vi "test_Set and Get 9475.vi"(8 "error in (no error)":errorcluster, 11 "TestCase in":refnum<class "Scan Engine Scripting API Custom Device Unit Tests.lvclass">) -> (0 "error out":errorcluster, 3 "TestCase out":refnum<class "Scan Engine Scripting API Custom Device Unit Tests.lvclass">)   [LabVIEW 2020, in "Scan Engine Scripting API Custom Device Unit Tests.lvclass"]
uses:
  Scan Engine Scripting API Custom Device Unit Tests.lvclass
  Scan Engine Scripting API Custom Device Unit Tests.lvclass/Scan Engine Scripting API Custom Device Unit Tests.ctl
  5525f2fe-c77f-4c69-8da2-db807206c7d6.vi
  Shared/Utility/Set Error.vi
  <vilib>/Utility/error.llb/Clear Errors.vi
  Scripting/Utility/Convert Slot Configuration to 9212.vi
  Scripting/Utility/Convert Slot Configuration to 9213.vi
  Scripting/Modules/NI 9475/NI 9475.lvclass
  C:/Users/nitest/Desktop/Git 2020/niveristand-scan-engine-ethercat-custom-device/Custom Device Source/Scripting/Modules/Module/Module.lvclass
  Includes/Modules.lvlibp/SD Module/SD Module.lvclass
  C:/Users/nitest/Desktop/Git 2020/niveristand-scan-engine-ethercat-custom-device/Includes/Modules.lvlibp/RSI Module/RSI Module.lvclass
  Scripting/Modules/NI 9212/NI 9212.lvclass
  Scripting/Modules/NI 9213/NI 9213.lvclass
  Scripting/Modules/NI 9224/NI 9224.lvclass
  Scripting/Modules/NI 9228/NI 9228.lvclass
  Includes/Modules.lvlibp/RSI Module/Read Module Page Property.vi
  Includes/Modules.lvlibp/RSI Module/Read Model.vi
  Scripting/Utility/Convert Module Model to Module Class.vi
  Includes/Modules.lvlibp/SD Module/Read DIO mode.vi
  Includes/Modules.lvlibp/RSI Module/Read Channels.vi
  Scripting/Utility/Convert to DI Module.vi
  Scripting/Utility/Convert to DO Module.vi
  Scripting/Utility/Convert to CI PWM Module.vi
  Scripting/Utility/Convert to CDO Module.vi
  Scripting/Utility/Convert to PWM Module.vi
  Shared/Globals/Error Strings.vi
  Scripting/Utility/Get Channel Names and Default Values for Slot.vi
  Scripting/Modules/NI 9212/Create NI 9212.vi
  Scripting/Modules/NI 9213/Create NI 9213.vi
  Scripting/Utility/Convert to AI Module.vi
  Scripting/Utility/Convert to AI Vrms Module.vi
  Scripting/Utility/Convert to AI Arms Module.vi
  Scripting/Utility/Convert to DIO Module.vi
  Scripting/Modules/Module/Module.lvclass
  Includes/Modules.lvlibp/9212/9212.lvclass
  Includes/Modules.lvlibp/9213/9213.lvclass
  Includes/Modules.lvlibp/9224/9224.lvclass
  <vilib>/addons/_JKI Toolkits/VI Tester/TestCase.llb/TestCase.lvclass
  Scripting/Scan Engine Scripting.lvlib
  C:/Program Files (x86)/National Instruments/LabVIEW 2020/vi.lib/addons/_JKI Toolkits/VI Tester/TestCase.llb/TestCase.lvclass
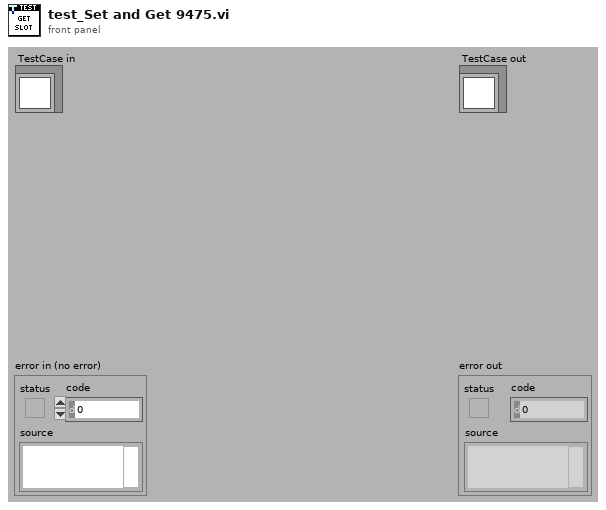
[diagram p1: front panel]
types:
  T1 = typedef "Custom Device API.lvlib/Custom Device Item Ref.ctl" = u64
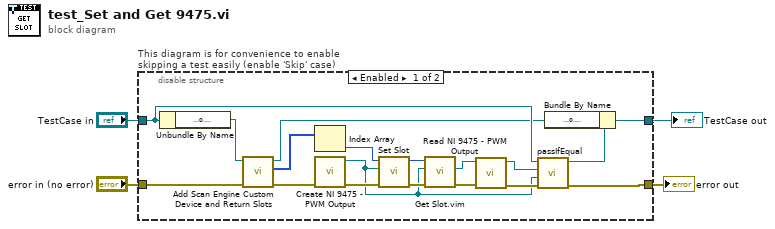
[diagram p0: block diagram]
diagram:
  n1 = disable-structure "This diagram is for convenience to enable skipping a test easily (enable 'Skip' case)" shown="Enabled" {
    disable-tunnel: "TestCase in" -> [w19 w26]
    disable-tunnel: [w21 w24] -> w1
    disable-tunnel: [w17 w25] -> w3
    disable-tunnel: "error in (no error)" -> [w10 w23]
    frame Enabled {
      n2 = Unbundle By Name(w19) -> ("target ref"=w12:refnum<k24>)
      n3 = call "Add Scan Engine Custom Device and Return Slots.vi"("error in"=w10, "target ref in"=w12) -> ("error out"=w9:errorcluster, "slot refs"=w11:T1[], "target ref out"=w8:refnum<k24>)  [unwired: 7 in]
      n4 = Index Array(array=w11) -> (element=w22:T1)  [unwired: 1 in]
      n5 = call "Create NI 9475 - PWM Output.vi"("error in"=w9) -> ("error out"=w18:errorcluster, "NI 9475 out"=w7:refnum<class "NI 9475.lvclass">)  [unwired: 9 in]
      n6 = call "Set Slot.vi"("error in"=w18, "module"=w7, "slot ref in"=w22) -> ("error out"=w20:errorcluster, "slot ref out"=w13:T1)  [unwired: 7 in]
      n7 = call "Get Slot.vim"("error in"=w20, "module type"=w7, "slot ref in"=w13) -> ("error out"=w5:errorcluster, "module"=w6:refnum<class "NI 9475.lvclass">)  [unwired: 5 in, 2 out]
      n8 = call "Read NI 9475 - PWM Output.vi"("error in (no error)"=w5, "NI 9475 in"=w6) -> ("error out"=w15:errorcluster, "NI 9475 out"=w16:refnum<class "NI 9475.lvclass">)  [unwired: 7 in, 1 out]
      n9 = call-dynamic "passIfEqual.vi"("error in (no error)"=w15, "y"=w7, "x"=w16, "TestCase in"=w19) -> ("error out"=w17:errorcluster, "TestCase out"=w14:refnum<class "Scan Engine Scripting API Custom Device Unit Tests.lvclass">)  [unwired: 6 in]
      n10 = Bundle By Name(cluster=w14, "target ref"=w8) -> (w21:refnum<class "Scan Engine Scripting API Custom Device Unit Tests.lvclass">)
    }
    frame Disabled {
      # "skip test result while test is under development"
      n11 = call <vilib>:"skip.vi"("error in (no error)"=w23, "TestCase in"=w26) -> ("error out"=w25:errorcluster, "TestCase out"=w24:refnum<class "Scan Engine Scripting API Custom Device Unit Tests.lvclass">)  [unwired: 8 in]
    }
  }
  "error out" <- w3
  "TestCase out" <- w1
